vi "GetImage.vi"(0 "XRef":T12, 1 "State In":T3) -> (14 "Image":T2, 15 "Fatal Error Out":T1)   [LabVIEW 2020, in "FlexBlock.xnode"]
uses:
  FlexBlock.xnode
  <vilib>/XNodeSupport/XNodeXNodeRef.ctl
  State.ctl
  FlexBlocks/Type Descriptor.ctl
  FlexBlocks/Terminal Direction.ctl
  FlexBlocks/Value Mode.ctl
  FlexBlocks/Terminal State.ctl
  FlexBlocks/Special Terminal.ctl
  FlexBlocks/Errors.ctl
  <vilib>/picture/picture.llb/imagedata.ctl
  FlexBlocks/Calculated Sizes.ctl
  <vilib>/XNodeSupport/XNodeImage.ctl
  <vilib>/XNodeSupport/XNodeErrorCluster.ctl
  <vilib>/XNodeSupport/NI_XNodeSupport.lvlib
  FlexBlocks/FlexBlocks.lvlib
panel:
  out "Full Picture":picture
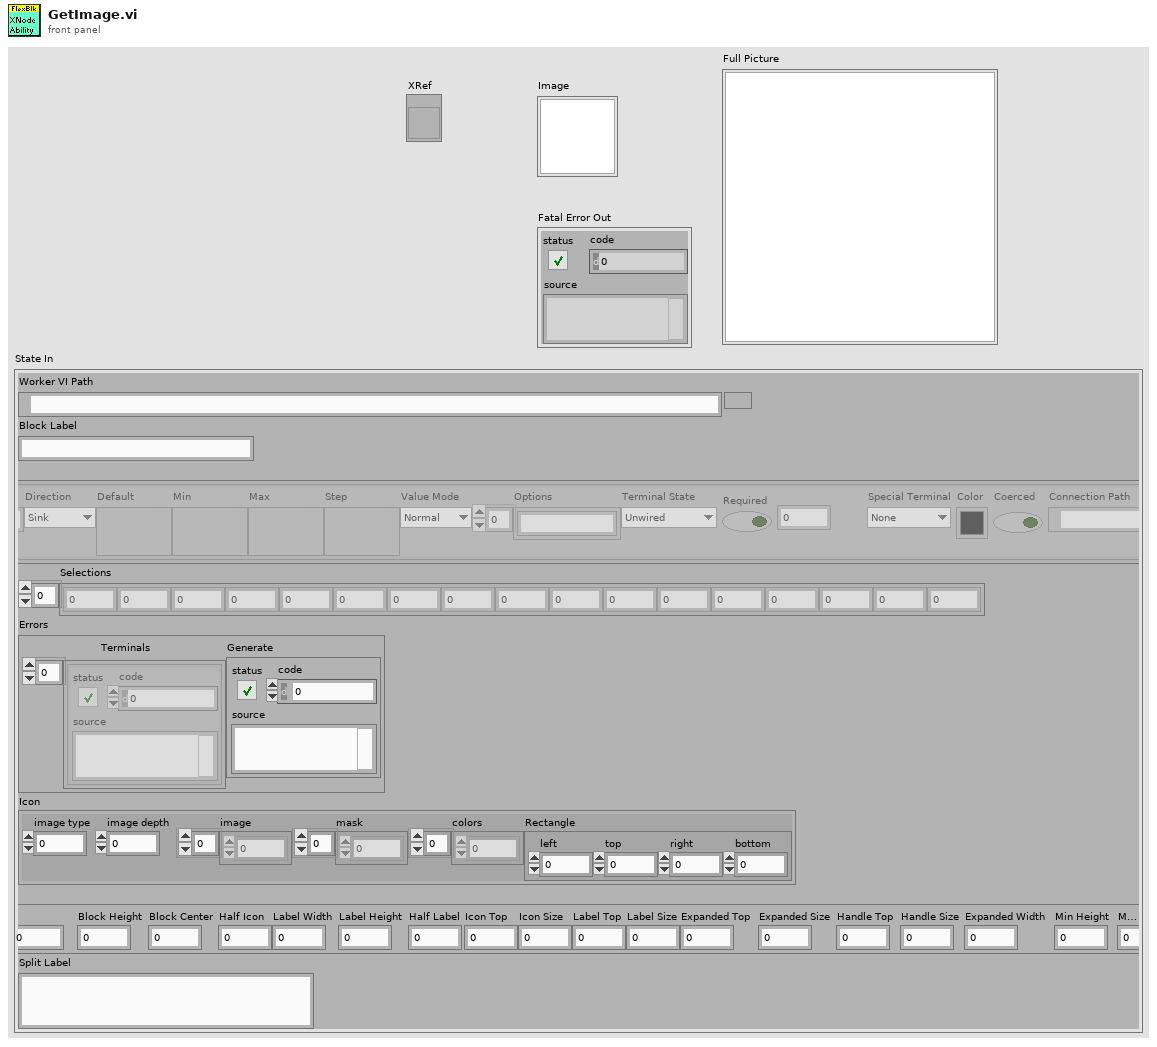
[diagram p1: front panel]
types:
  T1 = typedef "NI_XNodeSupport.lvlib/XNodeErrorCluster.ctl" = errorcluster
  T2 = typedef "NI_XNodeSupport.lvlib/XNodeImage.ctl" = picture
  T3 = typedef "FlexBlock.xnode/State.ctl" = cluster{"Worker VI Path":path, "Block Label":string, "Types":T4[], "Selections":i32[], "Errors":T9, "Icon":T10, "Calcd Sizes":T11, "Split Label":string}
  T4 = typedef "FlexBlocks.lvlib/Type Descriptor.ctl" = cluster{"Name":string, "Direction":T5, "Default":variant, "Min":variant, "Max":variant, "Step":variant, "Value Mode":T6, "Options":string[], "Terminal State":T7, "Required":bool, "Connpane Index":i32, "Special Terminal":T8, "Color":u32, "Coerced":bool, "Connection Path":path, "Draw Style":T7}
  T5 = typedef "FlexBlocks.lvlib/Terminal Direction.ctl" = enum16{"Sink", "Source"}
  T6 = typedef "FlexBlocks.lvlib/Value Mode.ctl" = enum16{"Normal", "Range", "Select"}
  T7 = typedef "FlexBlocks.lvlib/Terminal State.ctl" = enum16{"Unwired", "BadType", "BadRef", "Channel", "Value", "Control Ref"}
  T8 = typedef "FlexBlocks.lvlib/Special Terminal.ctl" = enum16{"None", "Action", "Init", "Tag", "State in", "State out", "Error"}
  T9 = typedef "FlexBlocks.lvlib/Errors.ctl" = cluster{"Terminals":errorcluster[], "Generate":errorcluster}
  T10 = typedef "imagedata.ctl" = cluster{"image type":i32, "image depth":i32, "image":u8[], "mask":u8[], "colors":u32[], "Rectangle":cluster{"left":i16, "top":i16, "right":i16, "bottom":i16}}
  T11 = typedef "FlexBlocks.lvlib/Calculated Sizes.ctl" = cluster{"Text Width":i32, "Text Height":i32, "Half Text":i32, "Block Width":i32, "Block Height":i32, "Block Center":i32, "Half Icon":i32, "Label Width":i32, "Label Height":i32, "Half Label":i32, "Icon Top":i32, "Icon Size":i32, "Label Top":i32, "Label Size":i32, "Expanded Top":i32, "Expanded Size":i32, "Handle Top":i32, "Handle Size":i32, "Expanded Width":i32, "Min Height":i32, "Max Height":i32}
  T12 = typedef "NI_XNodeSupport.lvlib/XNodeXNodeRef.ctl" = refnum<vi>
  T13 = typedef "FlexBlocks.lvlib/Size Constants.ctl" = cluster{"Icon":i32, "Value Width":i32, "BG Rounding":i32, "Term Width":i32, "Term Height":i32, "Text Offset":i32, "Value Padding":i32, "Select Padding":i32, "Min Block Width":i32, "Vertical Margin":i32, "Size Handle Height":i32, "Name Padding":i32, "Collapsed Spacing":i32}
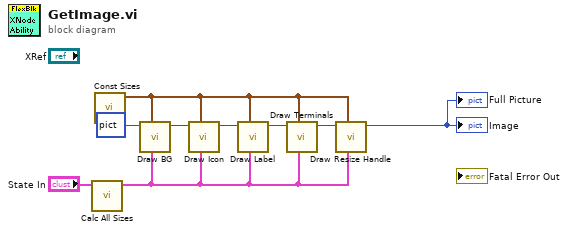
[diagram p0: block diagram]
diagram:
  n1 = call "Calc All Sizes.vi"("State In"="State In") -> ("State"=w1:T3)  [unwired: 10 in]
  n2 = call "Const Sizes.vi"() -> ("Sizes"=w4:T13)  [unwired: 11 in]
  n3 = call "Draw BG.vi"("State"=w1, "Sizes"=w4, "Picture  In"=picture data[5B]) -> ("Picture"=w8:picture)  [unwired: 8 in]
  n4 = call "Draw Icon.vi"("State"=w1, "Sizes"=w4, "Picture  In"=w8) -> ("Picture"=w7:picture)  [unwired: 8 in]
  n5 = call "Draw Label.vi"("State"=w1, "Sizes"=w4, "Picture  In"=w7) -> ("Picture"=w6:picture)  [unwired: 8 in]
  n6 = call "Draw Terminals.vi"("State"=w1, "Sizes"=w4, "Picture  In"=w6) -> ("Picture"=w5:picture)  [unwired: 8 in]
  n7 = call "Draw Resize Handle.vi"("State"=w1, "Sizes"=w4, "Picture  In"=w5) -> ("Picture"=→"Image" →"Full Picture":picture)  [unwired: 8 in]
